vi "main_program.vi"() -> ()   [LabVIEW 2020]
uses:
  <vilib>/Instr/_visa.llb/VISA Configure Serial Port (Instr).vi
panel:
  in  "Sampling rate in values / sec":dbl=1000.0
  in  "Sensor":tag="SimDev1/ai0:1"
  in  "Select":bool
  in  "Select the program":u16(ring) items=["Adjustment ", "Tensile test", "Exit"]
  in  "VISA resource name":refnum<visa-resource-name>
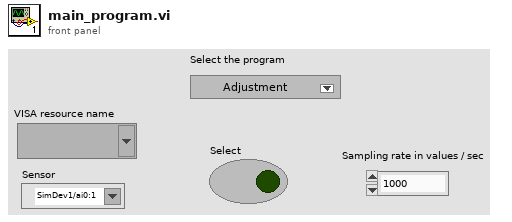
[diagram p1: front panel]
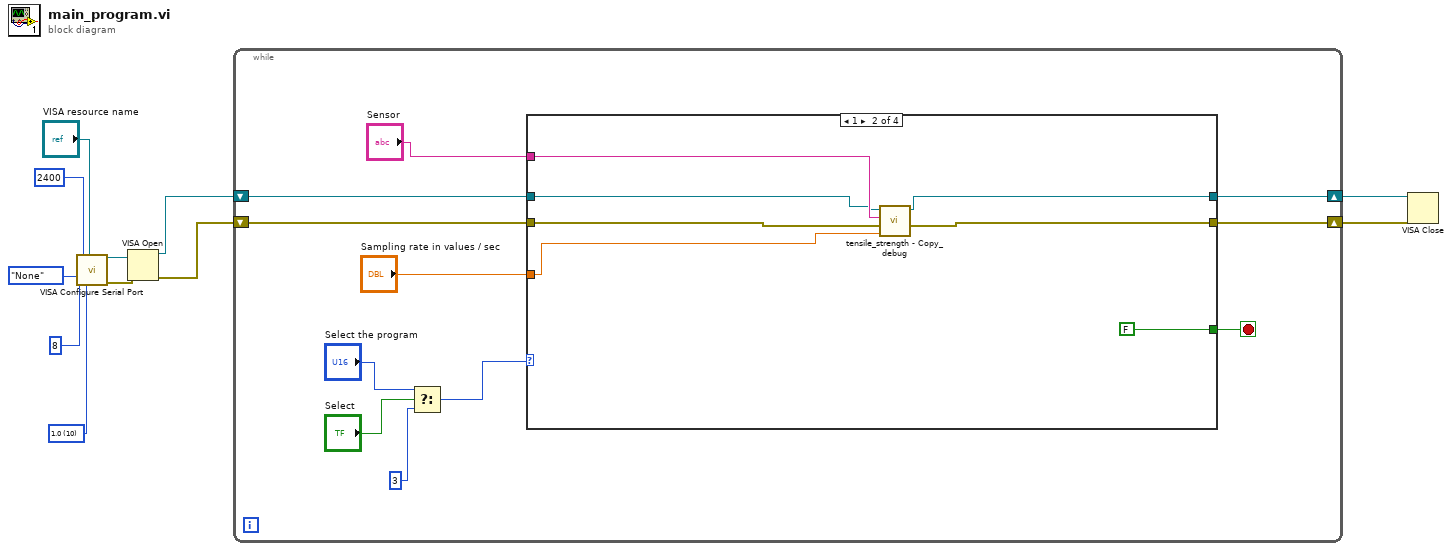
[diagram p0: block diagram]
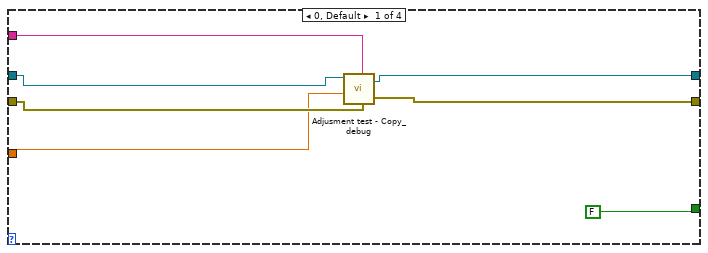
[diagram p2: hidden frame]
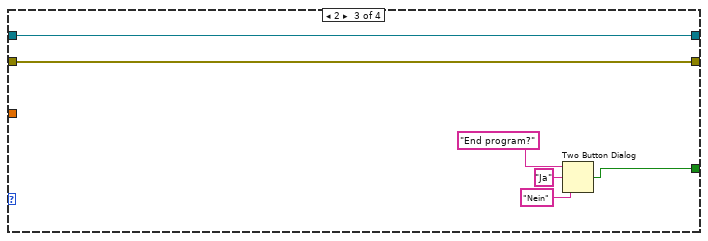
[diagram p3: hidden frame]
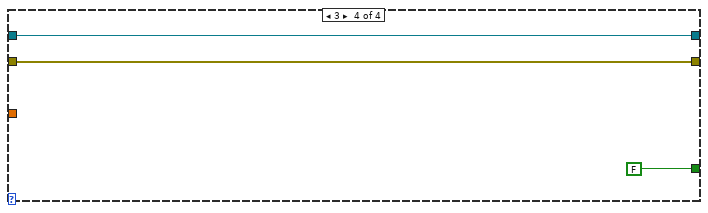
[diagram p4: hidden frame]
diagram:
  w1 = u16 10 items=["1.0"=10, "1.5"=15, "2.0"=20] ("stop bits (10: 1 bit)")
  n1 = call-poly "VISA Configure Serial Port"("VISA resource name"="VISA resource name", "baud rate (9600)"=u32 2400, "data bits (8)"=u16 8, "parity (0:none)"=enum16{"None", "Odd", "Even", "Mark", "Space"}."None", "stop bits (10: 1 bit)"=w1) -> ("VISA resource name out"=w7:refnum<visa-resource-name>, "error out"=w6:errorcluster)  [unwired: 9 in]
  n2 = VISA Open(error in (no error)=w6, VISA resource name=w7) -> (VISA resource name=w11:refnum<visa-resource-name>, error out=w10:errorcluster)  [unwired: 3 in]
  n3 = while {
    shift-right: [w19] -> w8
    shift-left: w11 -> [w22]
    shift-right: [w20] -> w9
    shift-left: w10 -> [w21]
    stop <- w13 stop-if-true
    n4 = Select(t="Select the program", s="Select", f=u16 3) -> (s? t:f=w15:u16)
    n5 = case shown="1" w15 {
      tunnel: w22 -> [w25 w32 w39 w45]
      tunnel: w21 -> [w24 w31 w38 w44]
      tunnel: [w27 w33 w38 w44] -> w20
      tunnel: [w28 w34 w39 w45] -> w19
      tunnel: "Sensor" -> [w26 w35 _ _]
      tunnel: [FALSE FALSE w37 FALSE] -> w13
      tunnel: "Sampling rate in values / sec" -> [w23 w30 _ _]
      frame 0, Default {
        n6 = call "Adjusment test - Copy_debug.vi"("error in (no error)"=w24, "Sampling rate"=w23, "Sensor"=w26, "VISA Refnum in"=w25) -> ("error out"=w27:errorcluster, "VISA Refnum out"=w28:refnum<visa-resource-name>)
      }
      frame 1 {
        n7 = call "tensile_strength - Copy_debug.vi"("Sampling rate"=w30, "error in (no error)"=w31, "Sensor"=w35, "VISA Refnum in"=w32) -> ("error out"=w33:errorcluster, "VISA Refnum out"=w34:refnum<visa-resource-name>)  [unwired: 6 in]
      }
      frame 2 {
        n8 = Two Button Dialog(message="End program?" ("Nachricht"), 1:"Nein" ("Text für F-Schaltfläche (\"Abbrechen\")"), 2:"Ja" ("Text für T-Schaltfläche (\"OK\")")) -> (T button?=w37:bool)
      }
      frame 3 {
      }
    }
  }
  n9 = VISA Close(VISA resource name=w8, error in (no error)=w9) -> ()  [unwired: 1 out]
